vi "RVC 4-link serial robot.vi"() -> ()   [LabVIEW 2013]
uses:
  <vilib>/robotics/Kinematics/DH Kinematic Parameters.ctl
  <vilib>/robotics/Kinematics/Link/Joint Type.ctl
  <vilib>/robotics/Kinematics/Robot/Robot Pose.ctl
  <vilib>/robotics/Kinematics/Analytical/Initialize Generic Serial Arm.vi
  <vilib>/robotics/Kinematics/Analytical/NI_Robotics_AnalyticKinematics.lvlib
  <vilib>/robotics/Kinematics/Link/NI_Robotics_Link.lvclass
  <vilib>/robotics/Kinematics/Robot/NI_Robotics_Serial Robot Arm.lvclass
panel:
  in  "joint positions":dbl[](array[slide])=[0.0, 0.0, 0.0, 0.0] scale=-3.0..3.0
  out "Array":T1[](array[typedef])
  out "transformation":picture
  in  "Pose":u16(ring) items=["qz", "qr", "qs", "qn", "free"]
  in  "stop":bool
  out "3D Picture":refnum<vi>(3d-picture)
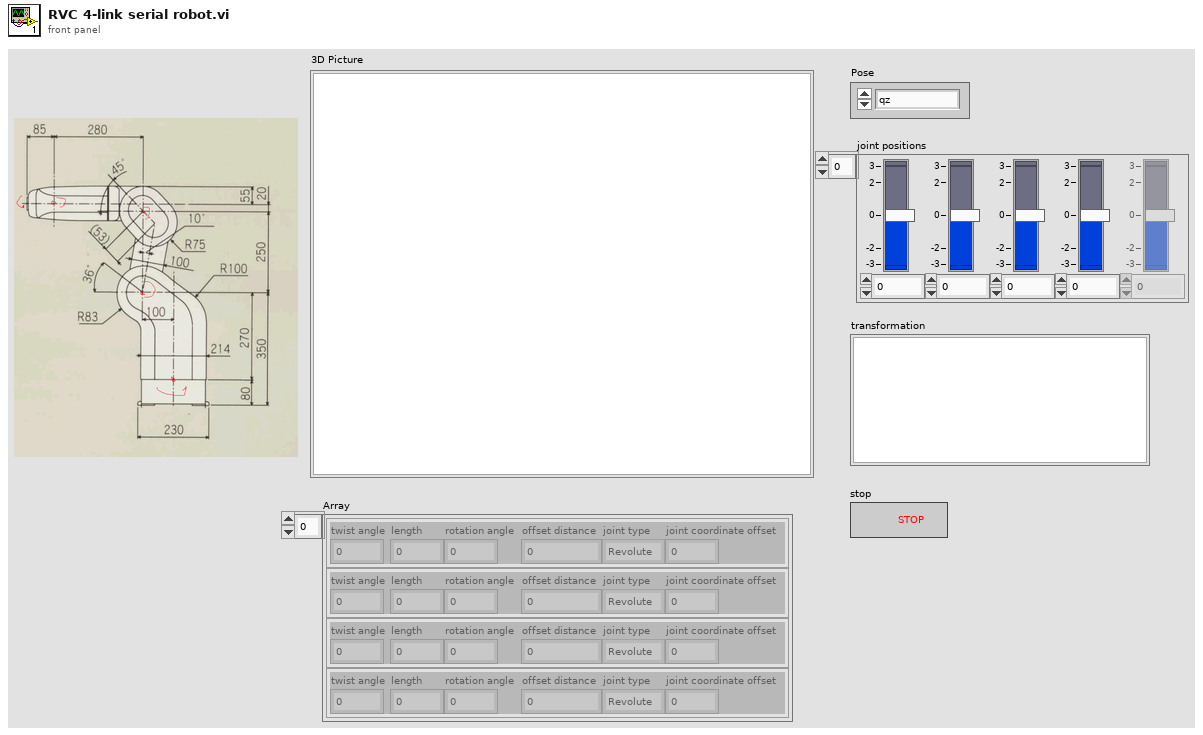
[diagram p1: front panel]
types:
  T1 = typedef "DH Kinematic Parameters.ctl" = cluster{"twist angle":dbl, "length":dbl, "rotation angle":dbl, "offset distance":dbl, "joint type":T2, "joint coordinate offset":dbl}
  T2 = typedef "NI_Robotics_Link.lvclass/Joint Type.ctl" = enum16{"Revolute", "Prismatic"}
  T3 = cluster{"Twist Angle":dbl, "Length":dbl, "Rotation Angle":dbl, "Offset Distance":dbl, "Joint Type":T2, "Joint Coordinate Offset":dbl}[]
  T4 = typedef "NI_Robotics_Serial Robot Arm.lvclass/Robot Pose.ctl" = cluster{"name":string, "description":string, "joint positions":dbl[]}
  T5 = typedef "NI_Matrix.lvlib/RealMatrix.ctl" = dbl[][]
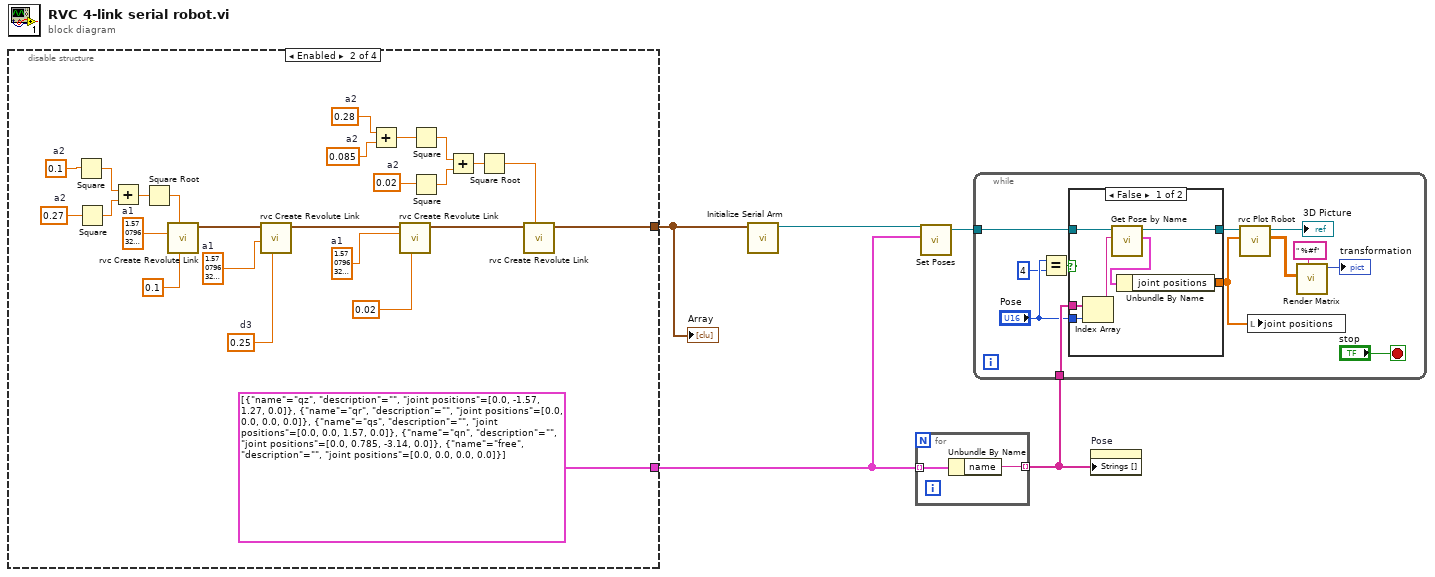
[diagram p0: block diagram]
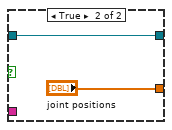
[diagram p2: hidden frame]
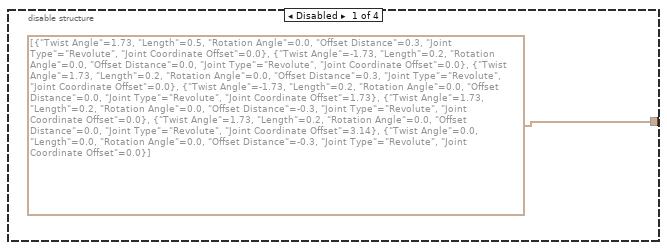
[diagram p3: hidden frame]
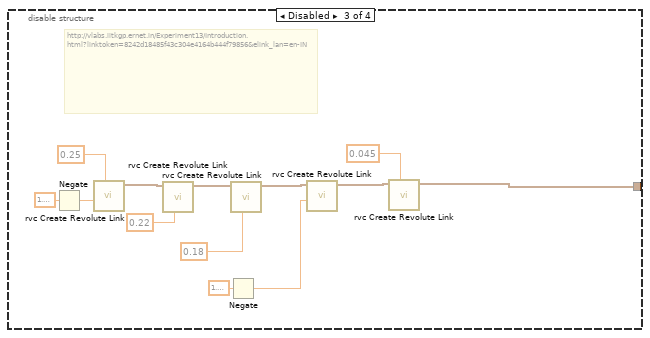
[diagram p4: hidden frame]
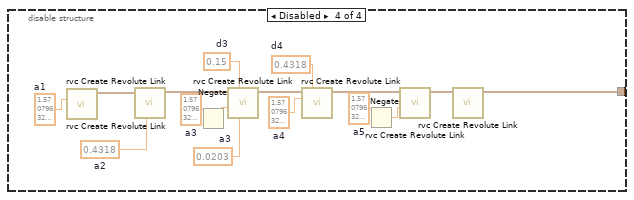
[diagram p5: hidden frame]
diagram:
  n1 = disable-structure shown="Enabled" {
    disable-tunnel: [T3 [{"Twist Angle"=1.73, "Length"=0.5, "Rotation Angle"=0.0, "Offset Distance"=0.3, "Joint Type"=enum."Revolute", "Joint Coordinate Offset"=0.0}, {"Twist Angle"=-1.73, "Length"=0.2, "Rotation Angle"=0.0, "Offset Distance"=0.0, "Joint Type"=enum."Revolute", "Joint Coordinate Offset"=0.0}, {"Twist Angle"=1.73, "Length"=0.2, "Rotation Angle"=0.0, "Offset Distance"=0.3, "Joint Type"=enum."Revolute", "Joint Coordinate Offset"=0.0}, {"Twist Angle"=-1.73, "Length"=0.2, "Rotation Angle"=0.0, "Offset Distance"=0.0, "Joint Type"=enum."Revolute", "Joint Coordinate Offset"=1.73}, {"Twist Angle"=1.73, "Length"=0.2, "Rotation Angle"=0.0, "Offset Distance"=-0.3, "Joint Type"=enum."Revolute", "Joint Coordinate Offset"=0.0}, {"Twist Angle"=1.73, "Length"=0.2, "Rotation Angle"=0.0, "Offset Distance"=0.0, "Joint Type"=enum."Revolute", "Joint Coordinate Offset"=3.14}, {"Twist Angle"=0.0, "Length"=0.0, "Rotation Angle"=0.0, "Offset Distance"=-0.3, "Joint Type"=enum."Revolute", "Joint Coordinate Offset"=0.0}] w16 w33 w59] -> w5
    disable-tunnel: [_ T4[] [{"name"="qz", "description"="", "joint positions"=[0.0, -1.57, 1.27, 0.0]}, {"name"="qr", "description"="", "joint positions"=[0.0, 0.0, 0.0, 0.0]}, {"name"="qs", "description"="", "joint positions"=[0.0, 0.0, 1.57, 0.0]}, {"name"="qn", "description"="", "joint positions"=[0.0, 0.785, -3.14, 0.0]}, {"name"="free", "description"="", "joint positions"=[0.0, 0.0, 0.0, 0.0]}] ("serial arm poses") _ _] -> w1
    frame Disabled {
    }
    frame Enabled {
      w11 = 1.5707963267948966  # a1
      w12 = 0.02  # a2
      w15 = 0.085  # a2
      w10 = 1.5707963267948966  # a1
      w14 = 0.28  # a2
      w27 = 0.27  # a2
      w21 = 1.5707963267948966  # a1
      w29 = 0.25  # d3
      w28 = 0.1  # a2
      n2 = Square(x=w28) -> (x^2=w25:dbl)
      n3 = Square(x=w27) -> (x^2=w26:dbl)
      n4 = Add(x=w25, y=w26) -> (x+y=w24:dbl)
      n5 = Square Root(x=w24) -> (sqrt(x)=w23:dbl)
      n6 = call "rvc Create Revolute Link.vi"("length (a)"=0.1 ("offset distance (d)"), "offset distance (d)"=w23, "twist angle (alpha)"=w21) -> ("Array"=w31:T1[])  [unwired: 8 in]
      n7 = call "rvc Create Revolute Link.vi"("length (a)"=w29, "joint coordinate offset"=w11, "Array 2"=w31) -> ("Array"=w30:T1[])  [unwired: 8 in]
      n8 = Add(x=w14, y=w15) -> (x+y=w13:dbl)
      n9 = call "rvc Create Revolute Link.vi"("length (a)"=0.02, "twist angle (alpha)"=w10, "Array 2"=w30) -> ("Array"=w17:T1[])  [unwired: 8 in]
      n10 = Square(x=w13) -> (x^2=w19:dbl)
      n11 = Square(x=w12) -> (x^2=w18:dbl)
      n12 = Add(x=w19, y=w18) -> (x+y=w20:dbl)
      n13 = Square Root(x=w20) -> (sqrt(x)=w9:dbl)
      n14 = call "rvc Create Revolute Link.vi"("offset distance (d)"=w9, "Array 2"=w17) -> ("Array"=w16:T1[])  [unwired: 9 in]
    }
    frame Disabled {
      # "http://vlabs.iitkgp.ernet.in/Experiment13/Introduction.html?linktoken=8242d18485f43c304e4164b444f79856&elink_lan=en-IN"
      n15 = Negate(x=1.5707963267948966 ("twist angle (alpha)")) -> (-x=w43:dbl)
      n16 = call "rvc Create Revolute Link.vi"("offset distance (d)"=0.25, "twist angle (alpha)"=w43) -> ("Array"=w41:T1[])  [unwired: 9 in]
      n17 = call "rvc Create Revolute Link.vi"("length (a)"=0.22, "Array 2"=w41) -> ("Array"=w39:T1[])  [unwired: 9 in]
      n18 = Negate(x=1.5707963267948966 ("twist angle (alpha)")) -> (-x=w35:dbl)
      n19 = call "rvc Create Revolute Link.vi"("length (a)"=0.18, "Array 2"=w39) -> ("Array"=w37:T1[])  [unwired: 9 in]
      n20 = call "rvc Create Revolute Link.vi"("twist angle (alpha)"=w35, "Array 2"=w37) -> ("Array"=w34:T1[])  [unwired: 9 in]
      n21 = call "rvc Create Revolute Link.vi"("offset distance (d)"=0.045, "Array 2"=w34) -> ("Array"=w33:T1[])  [unwired: 9 in]
    }
    frame Disabled {
      w46 = 1.5707963267948966  # a5
      w47 = 0.4318  # d4
      w48 = 1.5707963267948966  # a4
      w50 = 1.5707963267948966  # a3
      w51 = 0.15  # d3
      w52 = 0.0203  # a3
      w56 = 0.4318  # a2
      w58 = 1.5707963267948966  # a1
      n22 = call "rvc Create Revolute Link.vi"("twist angle (alpha)"=w58) -> ("Array"=w57:T1[])  [unwired: 10 in]
      n23 = call "rvc Create Revolute Link.vi"("length (a)"=w56, "Array 2"=w57) -> ("Array"=w55:T1[])  [unwired: 9 in]
      n24 = Negate(x=w50) -> (-x=w49:dbl)
      n25 = call "rvc Create Revolute Link.vi"("length (a)"=w52, "offset distance (d)"=w51, "twist angle (alpha)"=w49, "Array 2"=w55) -> ("Array"=w54:T1[])  [unwired: 7 in]
      n26 = call "rvc Create Revolute Link.vi"("offset distance (d)"=w47, "twist angle (alpha)"=w48, "Array 2"=w54) -> ("Array"=w53:T1[])  [unwired: 8 in]
      n27 = Negate(x=w46) -> (-x=w45:dbl)
      n28 = call "rvc Create Revolute Link.vi"("twist angle (alpha)"=w45, "Array 2"=w53) -> ("Array"=w60:T1[])  [unwired: 9 in]
      n29 = call "rvc Create Revolute Link.vi"("Array 2"=w60) -> ("Array"=w59:T1[])  [unwired: 10 in]
    }
  }
  "Array" <- w5
  n30 = call-poly <vilib>:"Initialize Serial Arm.vi"("kinematic parameters"=w5) -> ("serial arm out"=w2:refnum<class "NI_Robotics_Serial Robot Arm.lvclass">)  [unwired: 9 in, 1 out]
  n31 = for {
    tunnel: w1 -> [w62] mode=indexing
    tunnel: [w61] -> w3 mode=indexing
    n32 = Unbundle By Name(w62) -> ("name"=w61:string)
  }
  n33 = call <vilib>:"Set Poses.vi"("serial arm poses"=w1, "serial arm in"=w2) -> ("serial arm out"=w4:refnum<class "NI_Robotics_Serial Robot Arm.lvclass">)  [unwired: 8 in, 1 out]
  n34 = while {
    tunnel: w4 -> [w73]
    tunnel: w3 -> [w70]
    stop <- "stop" stop-if-true
    n35 = Equal?(x="Pose", y=u16 4) -> (x = y?=w64:bool)
    n36 = case shown="False" w64 {
      tunnel: w73 -> [w81 w83]
      tunnel: [w80 w83] -> w72
      tunnel: w70 -> [w79 _]
      tunnel: "Pose" -> [w77 _]
      tunnel: [w75 "joint positions"] -> w63
      frame False {
        n37 = Index Array(array=w79, index=w77) -> (element=w78:string)
        n38 = call <vilib>:"Get Pose by Name.vi"("name"=w78, "serial arm in"=w81) -> ("serial arm pose"=w76:T4, "serial arm out"=w80:refnum<class "NI_Robotics_Serial Robot Arm.lvclass">)  [unwired: 7 in, 1 out]
        n39 = Unbundle By Name(w76) -> ("joint positions"=w75:dbl[])
      }
      frame True {
      }
    }
    n40 = call "rvc Plot Robot.vi"("joint positions"=w63, "NI_Robotics_Serial Robot Arm in"=w72) -> ("forward kinematics"=w69:T5, "Scene Object Out"=→"3D Picture":refnum<vi>)  [unwired: 8 in]
    n41 = local write "joint positions"(w63) -> ()
    n42 = call "Render Matrix.vi"("format string"=" %#f", "A"=w69) -> ("picture out"=→"transformation":picture)  [unwired: 9 in]
  }
  n43 = property on="Pose" class="Ring (strict)"("Strings []"=w3) -> ()  [unwired: 2 in, 2 out]
